vi "Initialize with Switch Parameters Core.vi"(8 "error in (no error)":errorcluster, 10 "Switch Parameters in":refnum<class "Abstract Switch Init Parameters.lvclass">, 11 "Mock SLSC Switch Consumer in":refnum<class "Mock SLSC Switch Consumer.lvclass">) -> (0 "error out":errorcluster, 3 "Mock SLSC Switch Consumer out":refnum<class "Mock SLSC Switch Consumer.lvclass">)   [LabVIEW 2017, in "Mock SLSC Switch Consumer.lvclass"]
uses:
  Mock SLSC Switch Consumer.lvclass
  SLSC-Switch-Simulator/Includes/CDMessaging.lvlibp/Switch/Abstract Switch Init Parameters/Abstract Switch Init Parameters.lvclass
  Mock SLSC Switch Consumer.lvclass/Mock SLSC Switch Consumer.ctl
  SLSC Switch Consumer/SLSC Switch Consumer.lvclass
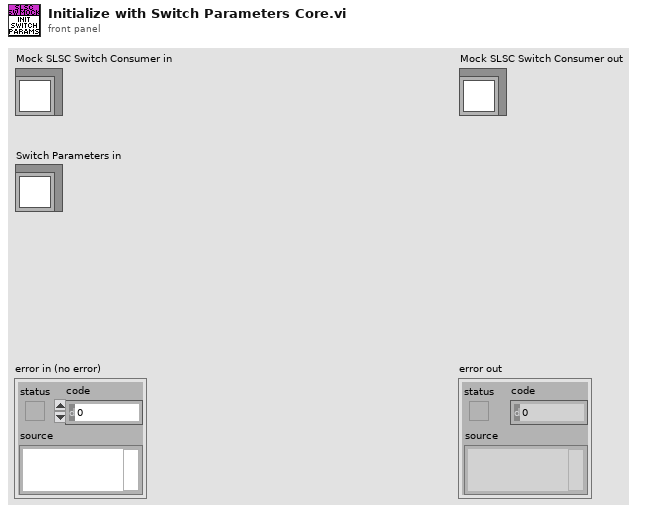
[diagram p1: front panel]
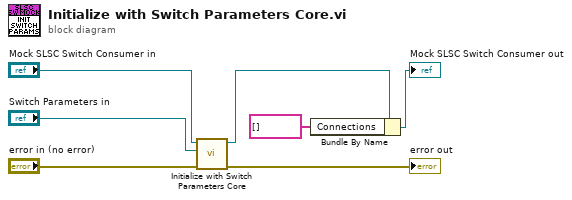
[diagram p0: block diagram]
diagram:
  n1 = call-parent "Initialize with Switch Parameters Core.vi"("error in (no error)"="error in (no error)", "Switch Parameters in"="Switch Parameters in", "SLSC Switch Consumer in"="Mock SLSC Switch Consumer in") -> ("error out"=→"error out":errorcluster, "SLSC Switch Consumer out"=w3:refnum<class "Mock SLSC Switch Consumer.lvclass">)  [unwired: 7 in]
  n2 = Bundle By Name(cluster=w3, "Connections"=string[] []) -> (→"Mock SLSC Switch Consumer out":refnum<class "Mock SLSC Switch Consumer.lvclass">)
